vi "Offset_decoder_with_sign_CH1.vi"(11 "Array In1":dbl[](array[numeric])) -> (2 "Sign CH1":dbl format="%.2f", 3 "CH1 SHIFT":dbl)   [LabVIEW 2012]
panel:
  # "1"
  # "CH0 LB"
  # "2"
  # "CH0 HB"
  # "3"
  # "CH0 UB"
  # "4"
  # "5"
  # "CH0 MB"
  # "CH0 sign"
  # "6"
  # "CH1 LB"
  # "7"
  # "CH1 HB"
  # "CH1 UB"
  # "CH1 MB"
  # "CH1 sign"
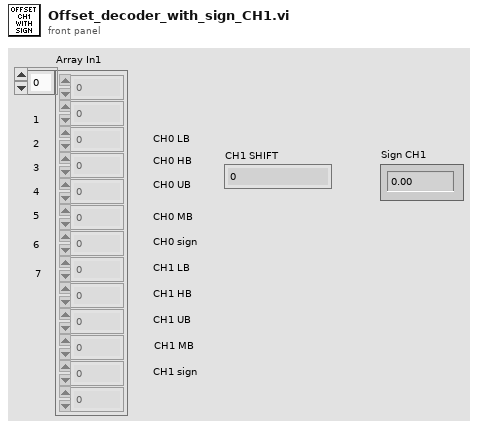
[diagram p1: front panel]
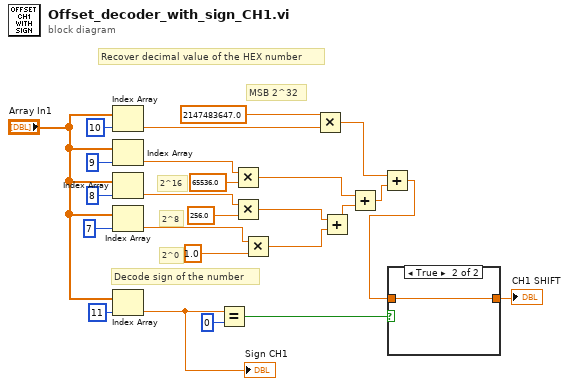
[diagram p0: block diagram]
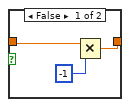
[diagram p2: hidden frame]
diagram:
  # "Decode sign of the number"
  # "Recover decimal value of the HEX number"
  # "2^0"
  # "2^8"
  # "2^16"
  # "MSB 2^32"
  n1 = Index Array(array="Array In1", index=10) -> (element=w1:dbl)
  n2 = Index Array(array="Array In1", index=9) -> (element=w16:dbl)
  n3 = Index Array(array="Array In1", index=8) -> (element=w18:dbl)
  n4 = Index Array(array="Array In1", index=7) -> (element=w20:dbl)
  n5 = Index Array(array="Array In1", index=11) -> (element=w2:dbl)
  "Sign CH1" <- w2
  n6 = Equal?(x=w2, y=0) -> (x = y?=w8:bool)
  n7 = Multiply(x=w16, y=65536.0) -> (x*y=w12:dbl)
  n8 = Multiply(x=w18, y=256.0) -> (x*y=w15:dbl)
  n9 = Multiply(x=w20, y=1.0) -> (x*y=w14:dbl)
  n10 = Multiply(x=2147483647.0, y=w1) -> (x*y=w4:dbl)
  n11 = Add(x=w15, y=w14) -> (x+y=w13:dbl)
  n12 = Add(x=w12, y=w13) -> (x+y=w11:dbl)
  n13 = Add(x=w4, y=w11) -> (x+y=w6:dbl)
  n14 = case shown="True" w8 {
    tunnel: w6 -> [w26 w29]
    tunnel: [w28 w29] -> w5
    frame False {
      n15 = Multiply(x=w26, y=-1) -> (x*y=w28:dbl)
    }
    frame True {
    }
  }
  "CH1 SHIFT" <- w5
